vi "test_python_32bit_23Q1.vi"() -> ()   [LabVIEW 2023]
panel:
  out "module path":path
  out "return value":string
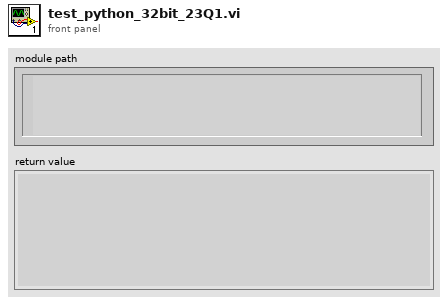
[diagram p1: front panel]
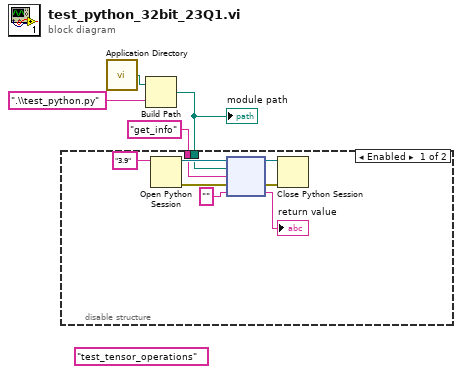
[diagram p0: block diagram]
diagram:
  (unwired) "test_tensor_operations" ("function name")
  n1 = call <vilib>:"Application Directory.vi"() -> ("Application Directory"=w3:path)
  n2 = Build Path(base path=w3, name or relative path=".\\test_python.py") -> (appended path=w1:path)
  "module path" <- w1
  n3 = disable-structure shown="Enabled" {
    disable-tunnel: "get_info" ("function name") -> [w8 _]
    disable-tunnel: w1 -> [w5 _]
    frame Enabled {
      n4 = Open Python Session(python version="3.9" ("Python version")) -> (session out=w13:refnum<k35>, error out=w12:errorcluster)  [unwired: 2 in]
      n5 = node(w13, w5, w8, w12, "" ("Python version")) -> (w11:refnum<k35>, w10:errorcluster, →"return value":string)  [unwired: 2 out]
      n6 = Close Python Session(session in=w11, error in=w10) -> ()  [unwired: 1 out]
    }
    frame Disabled {
    }
  }
